vi "read refnum.vi"(6 "call chain index (1)":i32=1, 7 "vi ref (caller)":refnum<vi>, 8 "error in (no error)":errorcluster, 11 "label":string) -> (0 "error out":errorcluster, 3 "refnum":refnum<vi>)   [LabVIEW 2024, in "controls manager.lvlib"]
uses:
  controls manager.lvlib
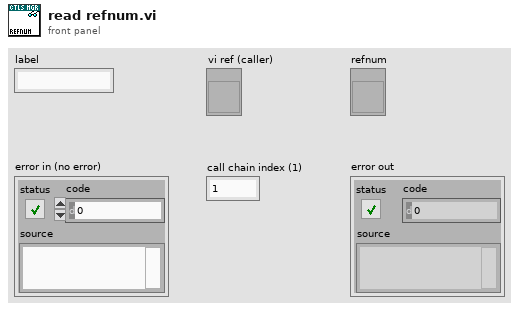
[diagram p1: front panel]
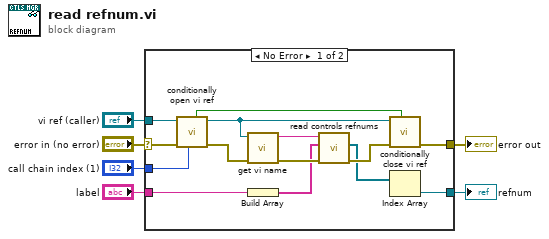
[diagram p0: block diagram]
diagram:
  n1 = case shown="No Error" "error in (no error)" {
    selector: "error in (no error)" -> [w19 w21]
    tunnel: [w16 w21] -> w6
    tunnel: "vi ref (caller)" -> [w13 _]
    tunnel: "call chain index (1)" -> [w12 _]
    tunnel: "label" -> [w11 _]
    tunnel: [w7 _] -> w1
    frame No Error {
      n2 = call "conditionally open vi ref.vi"("call chain index (1)"=w12, "error in (no error)"=w19, "vi ref in"=w13) -> ("error out"=w18:errorcluster, "vi ref out"=w10:refnum<vi>, "new ref?"=w15:bool)  [unwired: 6 in]
      n3 = call "get vi name.vi"("error in (no error)"=w18, "vi ref"=w10) -> ("error out"=w20:errorcluster, "vi name"=w14:string)  [unwired: 8 in]
      n4 = Build Array(w11) -> (w9:string[])
      n5 = call "read controls refnums.vi"("error in (no error)"=w20, "labels"=w9, "id"=w14) -> ("error out"=w17:errorcluster, "refnums"=w8:refnum<vi>[])  [unwired: 7 in]
      n6 = call "conditionally close vi ref.vi"("new ref?"=w15, "error in (no error)"=w17, "vi ref"=w10) -> ("error out"=w16:errorcluster)  [unwired: 8 in]
      n7 = Index Array(array=w8) -> (element=w7:refnum<vi>)  [unwired: 1 in]
    }
    frame Error {
    }
  }
  "error out" <- w6
  "refnum" <- w1
